vi "ARC_Queue Destroy_Array.vi"(8 "error in (no error)":errorcluster caption="Error In (no error)", 11 "Queue name":string[](array[string])) -> (0 "error out":errorcluster caption="Error Out", 2 "Remaining Elements":cluster{"Event":string, "Data":variant}[][](array[cluster]), 3 "Queue Name":string[](array[string]))   [LabVIEW 2016]
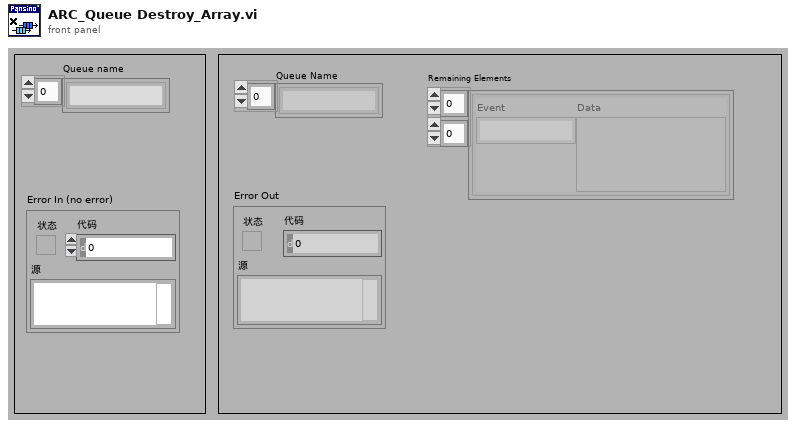
[diagram p1: front panel]
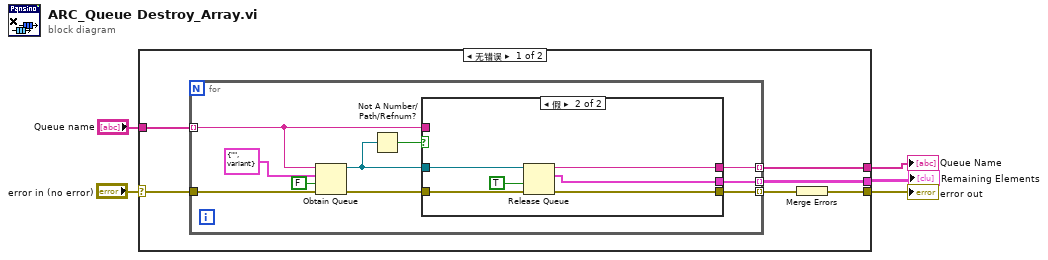
[diagram p0: block diagram]
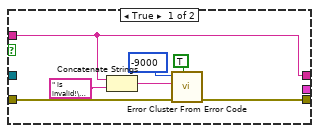
[diagram p2: hidden frame]
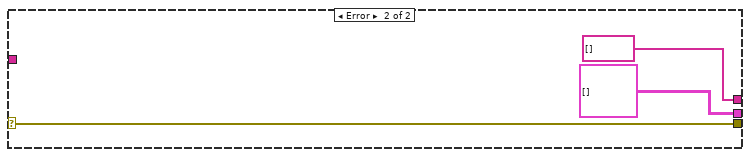
[diagram p3: hidden frame]
diagram:
  n1 = case shown="无错误" "error in (no error)" {
    selector: "error in (no error)" -> [w10 w37]
    tunnel: [w9 w37] -> w5
    tunnel: "Queue name" -> [w8 _]
    tunnel: [w7 string[] []] -> w2
    tunnel: [w6 cluster{"Event":string, "Data":variant}[][] [] ("remaining elements")] -> w1
    frame No Error {
      n2 = for {
        tunnel: w8 -> [w13] mode=indexing
        tunnel: [w21] -> w11 mode=indexing
        tunnel: [w20] -> w7 mode=indexing
        tunnel: [w19] -> w6 mode=indexing
        tunnel: w10 -> [w17]
        n3 = Obtain Queue(name (unnamed)=w13, element data type=cluster{"Event":string, "Data":variant} {"Event"="", "Data"=variant} ("输出簇"), create if not found? (T)=FALSE ("如未找到是否创建？(T)"), error in (no error)=w17) -> (queue out=w15:refnum<queue>, error out=w14:errorcluster)  [unwired: 1 in, 1 out]
        n4 = Not A Number/Path/Refnum?(number/path/refnum=w15) -> (NaN/Path/Refnum?=w16:bool)
        n5 = case shown="假" w16 {
          tunnel: [w24 w32] -> w21
          tunnel: w14 -> [w25 w33]
          tunnel: [w23 w31] -> w20
          tunnel: [_ w30] -> w19
          tunnel: w15 -> [_ w34]
          tunnel: w13 -> [w23 _]
          frame True {
            n6 = Concatenate Strings(w23, " is invalid!\nEnsure the queue has been created!" ("字符串")) -> (w26:string)
            n7 = call <vilib>:"Error Cluster From Error Code.vi"("show call chain? (False)"=TRUE, "error in (no error)"=w25, "error message (\"\")"=w26, "error code (0)"=-9000) -> ("error out"=w24:errorcluster)  [unwired: 5 in]
          }
          frame False {
            n8 = Release Queue(queue=w34, force destroy? (F)=TRUE ("强制销毁？(F)"), error in (no error)=w33) -> (queue name=w31:string, remaining elements=w30:cluster{"Event":string, "Data":variant}[], error out=w32:errorcluster)
          }
        }
      }
      n9 = Merge Errors(w11) -> (w9:errorcluster)
    }
    frame Error {
    }
  }
  "error out" <- w5
  "Queue Name" <- w2
  "Remaining Elements" <- w1
